vi "inerpretar error.vi"(11 "error out":errorcluster) -> (0 "Alarma Proximidad Encoder":bool, 1 "Alarma Proximidad MOtor":bool, 2 "Alarma Final Carrera Motor":bool, 3 "Alarma Driver":bool, 4 "Alarma Final Carrea Encoder":bool, 6 "Alarma No es un numero":bool)   [LabVIEW 2011]
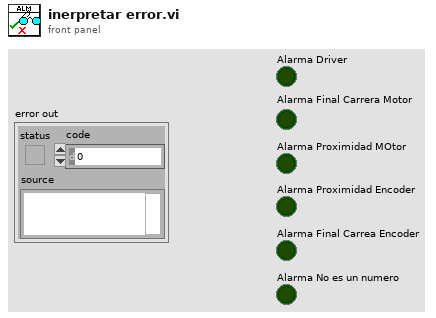
[diagram p1: front panel]
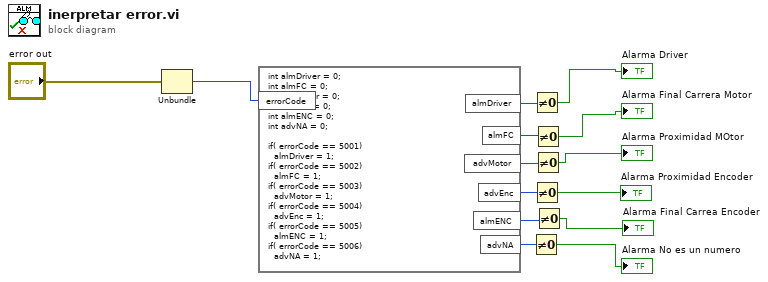
[diagram p0: block diagram]
diagram:
  n1 = Unbundle("error out") -> ("code"=w13:i32)  [unwired: 2 out]
  n2 = formula code="int almDriver = 0;\nint almFC = 0;\nint advMotor = 0;\nint advEnc = 0;\nint almENC = 0;\nint advNA = 0;\n\nif( errorCode == 5001)\n  almDriver = 1;\nif( errorCode == 5002)\n  almFC = 1;\nif( errorCode == 5003)\n  advMotor = 1;\nif( errorCode == 5004)\n  advEnc = 1;\nif( errorCode == 5005)\n  almENC = 1;\nif( errorCode == 5006)\n  advNA = 1;"("errorCode"=w13) -> ("almDriver"=w12:i32, "almFC"=w11:i32, "advMotor"=w10:i32, "advEnc"=w9:i32, "advNA"=w8:i32, "almENC"=w2:i32)
  n3 = Not Equal To 0?(x=w8) -> (x != 0?=→"Alarma No es un numero":bool)
  n4 = Not Equal To 0?(x=w12) -> (x != 0?=→"Alarma Driver":bool)
  n5 = Not Equal To 0?(x=w9) -> (x != 0?=→"Alarma Proximidad Encoder":bool)
  n6 = Not Equal To 0?(x=w11) -> (x != 0?=→"Alarma Final Carrera Motor":bool)
  n7 = Not Equal To 0?(x=w10) -> (x != 0?=→"Alarma Proximidad MOtor":bool)
  n8 = Not Equal To 0?(x=w2) -> (x != 0?=→"Alarma Final Carrea Encoder":bool)
